vi "SonifyGlobals.vi"() -> ()   [LabVIEW 2016]
panel:
  in  "File Path":path=path "C:/Data/Sonify Labview/ChickenWithChillerWithStandoff.lvm" caption="Filename"
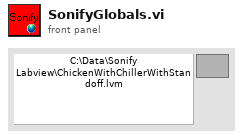
[diagram p1: front panel]
diagram:
